vi "color-detection(SubVI).vi"(4 "Cube Blue":dbl, 6 "Cube Green":dbl, 7 "Box Red":dbl, 9 "Cube Red":dbl, 10 "Box Blue":dbl, 11 "Box Green":dbl) -> (2 "COLOR CUBE":dbl, 3 "COLOR BOX":dbl)   [LabVIEW 2016]
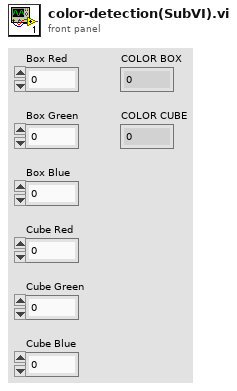
[diagram p1: front panel]
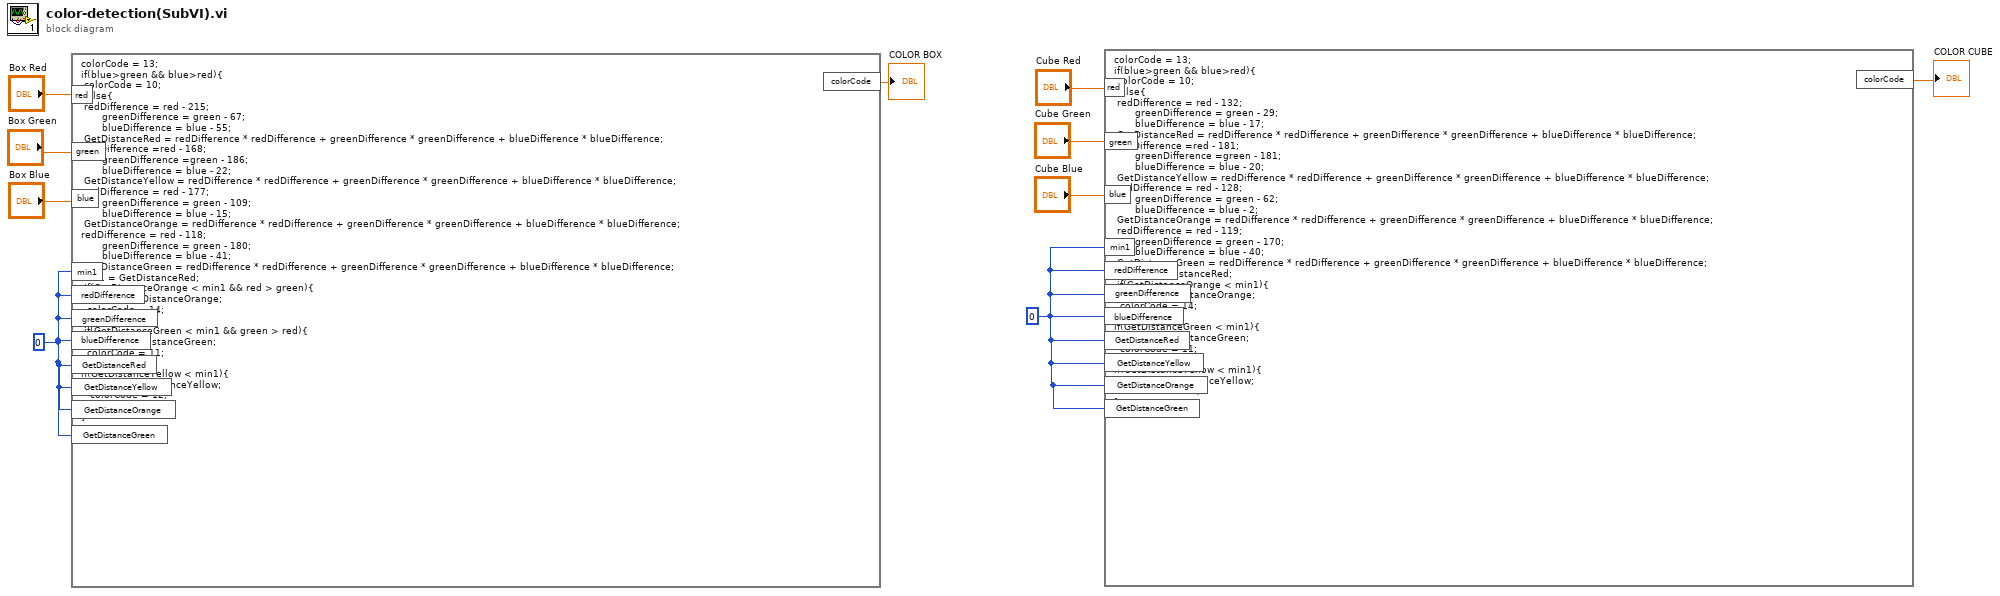
[diagram p0: block diagram]
diagram:
  w10 = 0
  w9 = 0
  n1 = formula code="colorCode = 13;\nif(blue>green && blue>red){\n\tcolorCode = 10;\n}else{\n\tredDifference = red - 215;\n       greenDifference = green - 67;\n       blueDifference = blue - 55;\n\tGetDistanceRed = redDifference * redDifference + greenDifference * greenDifference + blueDifference * blueDifference;\n\tredDifference =red - 168;\n       greenDifference =green - 186;\n       blueDifference = blue - 22;\n\tGetDistanceYellow = redDifference * redDifference + greenDifference * greenDifference + blueDifference * blueDifference;\n\tredDifference = red - 177;\n       greenDifference = green - 109;\n       blueDifference = blue - 15;\n\tGetDistanceOrange = redDifference * redDifference + greenDifference * greenDifference + blueDifference * blueDifference;\nredDifference = red - 118;\n       greenDifference = green - 180;\n       blueDifference = blue - 41;\n\tGetDistanceGreen = redDifference * redDifference + greenDifference * greenDifference + blueDifference * blueDifference;\t\nmin1 = GetDistanceRed;\n\tif(GetDistanceOrange < min1 && red > green){\n\t\tmin1 = GetDistanceOrange;\n\t\tcolorCode = 14;\n\t}\n\tif(GetDistanceGreen < min1 && green > red){\n\t\tmin1 = GetDistanceGreen;\n\t\tcolorCode = 11;\n\t}\nif(GetDistanceYellow < min1){\n\t\t\tmin1 = GetDistanceYellow;\n\t\t colorCode = 12;\n}\n}"("red"="Box Red", "blue"="Box Blue", "green"="Box Green", "redDifference"=w9, "greenDifference"=w9, "blueDifference"=w9, "GetDistanceRed"=w9, "GetDistanceYellow"=w9, "GetDistanceOrange"=w9, "min1"=w9, "GetDistanceGreen"=w9) -> ("colorCode"=→"COLOR BOX":dbl)
  n2 = formula code="colorCode = 13;\nif(blue>green && blue>red){\n\tcolorCode = 10;\n}else{\n\tredDifference = red - 132;\n       greenDifference = green - 29;\n       blueDifference = blue - 17;\n\tGetDistanceRed = redDifference * redDifference + greenDifference * greenDifference + blueDifference * blueDifference;\n\tredDifference =red - 181;\n       greenDifference =green - 181;\n       blueDifference = blue - 20;\n\tGetDistanceYellow = redDifference * redDifference + greenDifference * greenDifference + blueDifference * blueDifference;\n\tredDifference = red - 128;\n       greenDifference = green - 62;\n       blueDifference = blue - 2;\n\tGetDistanceOrange = redDifference * redDifference + greenDifference * greenDifference + blueDifference * blueDifference;\n\tredDifference = red - 119;\n       greenDifference = green - 170;\n       blueDifference = blue - 40;\n\tGetDistanceGreen = redDifference * redDifference + greenDifference * greenDifference + blueDifference * blueDifference;\t\nmin1 = GetDistanceRed;\n\tif(GetDistanceOrange < min1){\n\t\tmin1 = GetDistanceOrange;\n\t\tcolorCode = 14;\n\t}\nif(GetDistanceGreen < min1){\n\t\tmin1 = GetDistanceGreen;\n\t\tcolorCode = 11;\n\t}\nif(GetDistanceYellow < min1){\n\t\t\tmin1 = GetDistanceYellow;\n\t\t colorCode = 12;\n}\n}"("red"="Cube Red", "blue"="Cube Blue", "green"="Cube Green", "redDifference"=w10, "greenDifference"=w10, "blueDifference"=w10, "GetDistanceRed"=w10, "GetDistanceYellow"=w10, "GetDistanceOrange"=w10, "min1"=w10, "GetDistanceGreen"=w10) -> ("colorCode"=→"COLOR CUBE":dbl)
